vi "program_log_sql.vi"() -> ()   [LabVIEW 2022 SP3]
panel:
  out "error out":errorcluster
  in  "OK Button":bool
  out "Starus":string
  in  "program":string(combo)
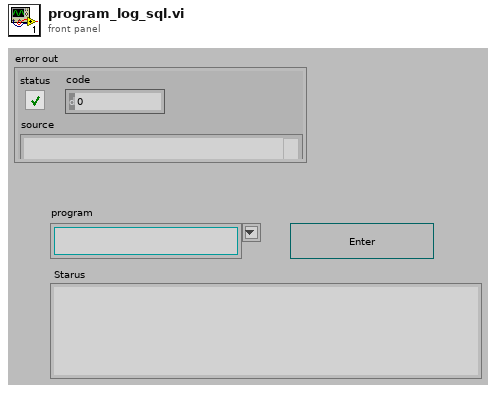
[diagram p1: front panel]
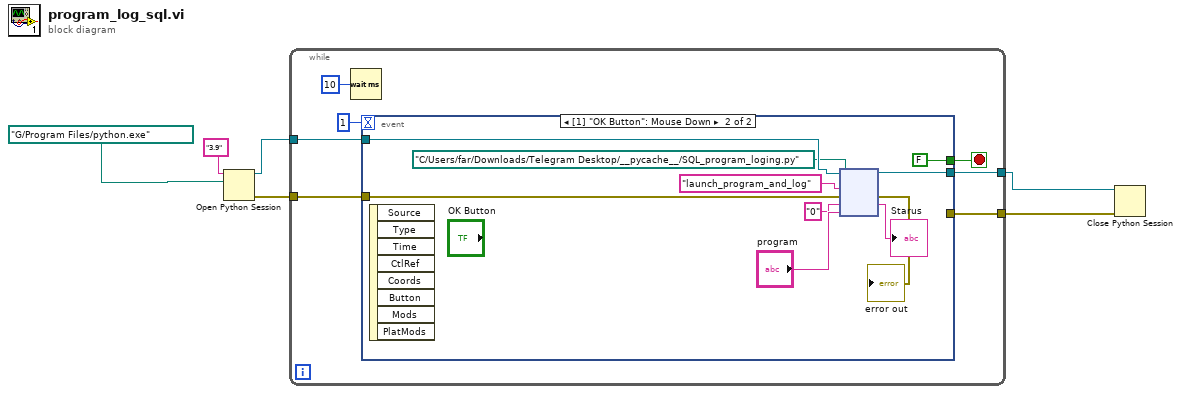
[diagram p0: block diagram]
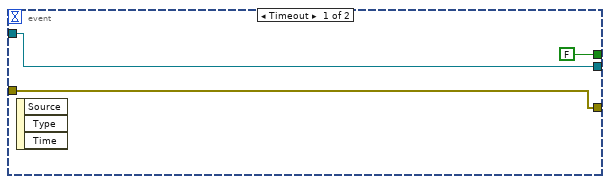
[diagram p2: hidden frame]
diagram:
  n1 = Open Python Session(python version="3.9" ("Python version"), python path=path "G:/Program Files/python.exe" ("Python path")) -> (session out=w5:refnum<k35>, error out=w4:errorcluster)  [unwired: 1 in]
  n2 = while {
    tunnel: [w13] -> w6
    tunnel: w5 -> [w9]
    tunnel: w4 -> [w8]
    tunnel: [w7] -> w1
    stop <- w12 stop-if-true
    n3 = Wait (ms)(milliseconds to wait=u32 10 ("millisecond timer value")) -> ()  [unwired: 1 out]
    n4 = event shown="[1] \"OK Button\": Mouse Down" {
      selector: _ -> [_ _]
      dyn-events: _ -> [_ _]
      timeout: 1 -> [_ _]
      tunnel: [w15 w23] -> w13
      tunnel: [FALSE FALSE] -> w12
      tunnel: w9 -> [w15 w20]
      tunnel: w8 -> [w14 w19]
      tunnel: [w14 _] -> w7
      event Timeout {
        n5 = event-data() -> ()  [unwired: 1 in, 3 out]
      }
      event "OK Button": Mouse Down {
        n6 = event-data() -> ()  [unwired: 1 in, 8 out]
        n7 = node(w20, path "C:/Users/far/Downloads/Telegram Desktop/__pycache__/SQL_program_loging.py" ("module path"), "launch_program_and_log" ("function name"), w19, "0", "program") -> (w23:refnum<k35>, →"error out":errorcluster, →"Starus":string)  [unwired: 1 in, 2 out]
      }
    }
  }
  n8 = Close Python Session(session in=w6, error in=w1) -> ()  [unwired: 1 out]
